vi "Find Magnitude.vi"(1 "FFT {X}":cdb[][](array[numeric]) format="%.2f") -> (0 "Magnitude":dbl[][](array[numeric]) format="%.2f")   [LabVIEW 2024]
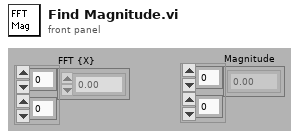
[diagram p1: front panel]
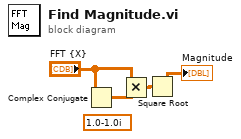
[diagram p0: block diagram]
diagram:
  (unwired) cdb 1.0-1.0i
  n1 = Complex Conjugate(1:"FFT {X}") -> (0:w1:cdb[][])
  n2 = Multiply(x="FFT {X}", y=w1) -> (x*y=w3:cdb[][])
  n3 = Square Root(x=w3) -> (sqrt(x)=→"Magnitude":cdb[][])
